vi "Harness - Action.vi"(8 "error in (no error)":errorcluster, 10 "Action":string, 11 "Class":path=path "C:/git/labview-icon-editor/Sandbox/Class 2/_Class.lvclass") -> (0 "error out":errorcluster)   [LabVIEW 2021, in "_IconEditorInterface.lvlib" / "_IconEditorInterface.lvclass"]
uses:
  Custom plugin interface/_IconEditorInterface.lvclass
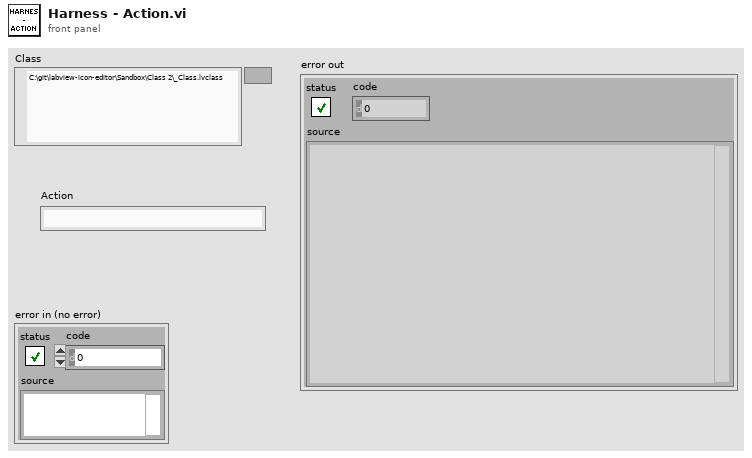
[diagram p1: front panel]
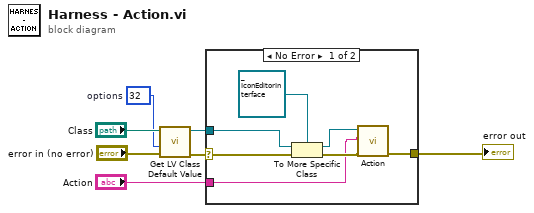
[diagram p0: block diagram]
diagram:
  w4 = u32 32  # options
  n1 = call <vilib>:"Get LV Class Default Value.vi"("error in (no error)"="error in (no error)", "options"=w4, "class path"="Class") -> ("error out"=w1:errorcluster, "object"=w7:refnum<class>)  [unwired: 7 in]
  n2 = case shown="No Error" w1 {
    selector: w1 -> [w8 w15]
    tunnel: w7 -> [w14 _]
    tunnel: [w12 w15] -> w3
    tunnel: "Action" -> [w11 _]
    frame No Error {
      n3 = To More Specific Class(target class=refnum<class "_IconEditorInterface.lvclass"> refnum ("_IconEditorInterface.lvlib:_IconEditorInterface.lvclass"), reference=w14, error in=w8) -> (specific class reference=w10:refnum<class "_IconEditorInterface.lvclass">, error out=w13:errorcluster)
      n4 = call-dynamic "Action.vi"("error in (no error)"=w13, "Action"=w11, "HarnessInterface in"=w10) -> ("error out"=w12:errorcluster)  [unwired: 7 in, 1 out]
    }
    frame Error {
    }
  }
  "error out" <- w3
